vi "例程51-动态波形幅值.vi"() -> ()   [LabVIEW 2016]
uses:
  <vilib>/measure/NI_MABase.lvlib
panel:
  in  "停止":bool
  out "波形图":waveform(dbl)(graph)
  in  "幅值":dbl=1.0 format="%0.2p"
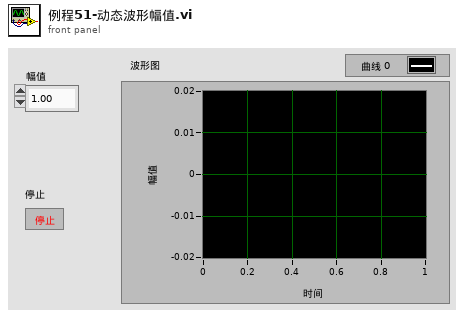
[diagram p1: front panel]
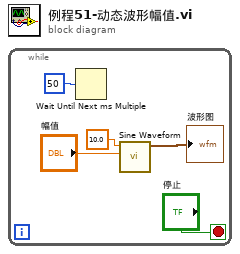
[diagram p0: block diagram]
diagram:
  n1 = while {
    stop <- "停止" stop-if-true
    n2 = Wait Until Next ms Multiple(millisecond multiple=u32 50 ("毫秒倍数")) -> ()  [unwired: 1 out]
    n3 = call <vilib>:"Sine Waveform.vi"("amplitude"="幅值", "frequency"=10.0) -> ("signal out"=→"波形图":waveform(dbl))  [unwired: 8 in, 1 out]
  }
